vi "sub_mr-timer.vi"(7 "cmd":enum16{"reset", "read"}(ring), 11 "limit s":u16=15) -> (2 "timeout":bool, 3 "time":dbl)   [LabVIEW 2018]
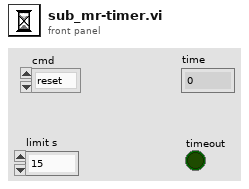
[diagram p1: front panel]
types:
  T1 = typedef "ctr-ref.ctl" = cluster{"connected":refnum<vi>, "start":refnum<vi>, "read_data":refnum<vi>, "Target":refnum<vi>, "play_type":refnum<vi>, "dt_daq":refnum<vi>, "dt_tcp":refnum<vi>, "timer":refnum<vi>, "States":refnum<vi>, "angle_limit":refnum<vi>, "Initial States":refnum<vi>}
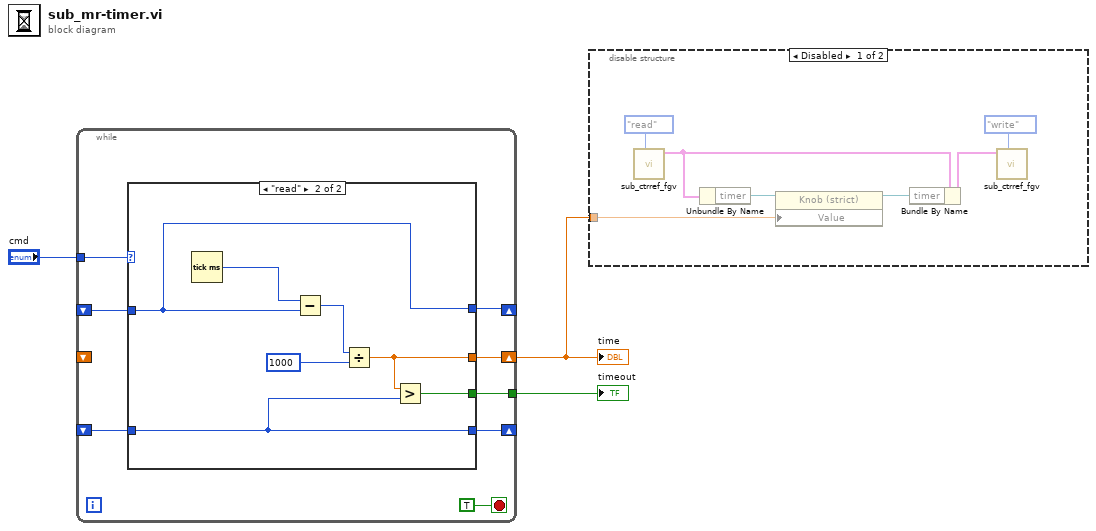
[diagram p0: block diagram]
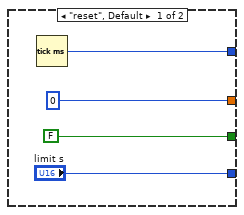
[diagram p3: hidden frame]
diagram:
  n1 = while {
    tunnel: "cmd" -> [w10]
    shift-right: [w9] -> w1
    shift-left: _ -> [_]
    shift-right: [w8] -> _
    shift-left: _ -> [w7]
    tunnel: [w6] -> w2
    shift-right: [w4] -> _
    shift-left: _ -> [w5]
    stop <- TRUE stop-if-true
    n2 = case shown="\"read\"" w10 {
      tunnel: [u16 0 w18] -> w9
      tunnel: w5 -> [_ w16]
      tunnel: [w14 w19] -> w8
      tunnel: w7 -> [_ w19]
      tunnel: [FALSE w17] -> w6
      tunnel: ["limit s" w16] -> w4
      frame "reset", Default {
        n3 = Tick Count (ms)() -> (millisecond timer value=w14:u32)
      }
      frame "read" {
        n4 = Tick Count (ms)() -> (millisecond timer value=w22:u32)
        n5 = Subtract(x=w22, y=w19) -> (x-y=w21:u32)
        n6 = Divide(x=w21, y=u32 1000) -> (x/y=w18:dbl)
        n7 = Greater?(x=w18, y=w16) -> (0:w17:bool)
      }
    }
  }
  "time" <- w1
  "timeout" <- w2
  n8 = disable-structure shown="Disabled" {
    disable-tunnel: w1 -> [w25 _]
    frame Disabled {
      n9 = call "sub_ctrref_fgv.vi"("cmd"=enum16{"write", "read"}."read") -> ("ctr_out"=w28:T1)  [unwired: 10 in]
      n10 = Unbundle By Name(w28) -> ("timer"=w27:refnum<vi>)
      n11 = property class="Knob (strict)"(reference=w27, "Value"=w25) -> (reference out=w26:refnum<vi>)  [unwired: 1 in, 1 out]
      n12 = Bundle By Name(cluster=w28, "timer"=w26) -> (w23:T1)
      n13 = call "sub_ctrref_fgv.vi"("cmd"=enum16{"write", "read"}."write", "ctr_in"=w23) -> ()  [unwired: 9 in, 1 out]
    }
    frame Enabled {
    }
  }
